vi "DBM Create Proc.vi"(8 "에러 입력":errorcluster, 11 "세부분류번호":string) -> (0 "에러 출력":errorcluster)   [LabVIEW 2020]
uses:
  Variables/Global_Constant.vi
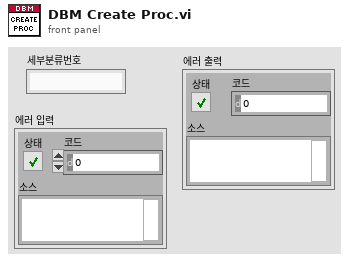
[diagram p1: front panel]
types:
  T1 = enum32{"Invalid", "Default", "Floating", "Floating/Auto-Hide", "Modal"}
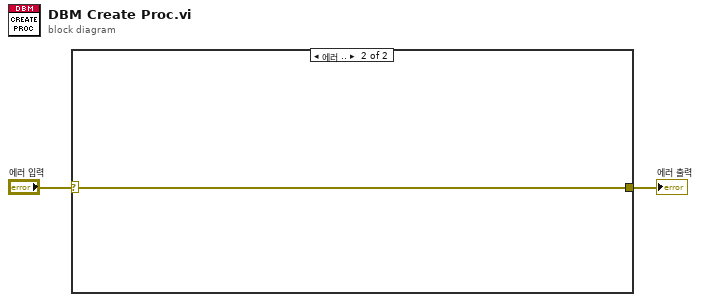
[diagram p0: block diagram]
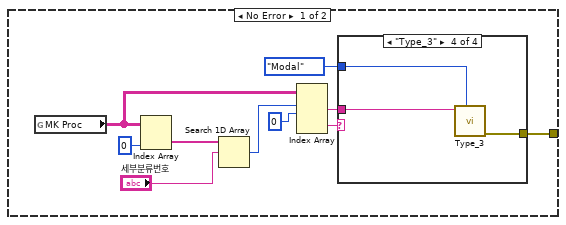
[diagram p2: hidden frame]
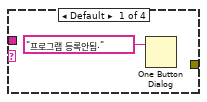
[diagram p3: hidden frame]
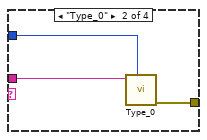
[diagram p4: hidden frame]
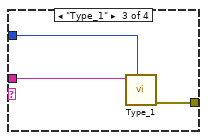
[diagram p5: hidden frame]
diagram:
  n1 = case shown="에러 .." "에러 입력" {
    selector: "에러 입력" -> [_ w23]
    tunnel: [w6 w23] -> w2
    frame No Error {
      n2 = global read "Global_Constant.vi" "MK Proc"() -> (w5:string[][])
      n3 = Index Array(array=w5, index (col)=0 ("비활성화된 인덱스 (열)")) -> (element=w11:string[])  [unwired: 1 in]
      n4 = Search 1D Array(1D array=w11, element="세부분류번호") -> (index of element=w9:i32)  [unwired: 1 in]
      n5 = Index Array(array=w5, index (row) #1=w9, index (col) #1=0 ("비활성화된 인덱스 (열)")) -> (element #1=w7:string, element #2=w4:string)  [unwired: 2 in]
      n6 = case shown="\"Type_3\"" w4 {
        tunnel: w7 -> [_ w16 w19 w22]
        tunnel: [_ w15 w18 w21] -> w6
        tunnel: T1."Modal" ("프런트패널 윈도우:동작") -> [_ w14 w17 w20]
        frame Default {
          n7 = One Button Dialog(message="프로그램 등록안됨." ("메시지")) -> ()  [unwired: 1 in, 1 out]
        }
        frame "Type_0" {
          n8 = call "Type_0.vi"("프런트패널 윈도우:동작"=w14, "세부분류코드"=w16) -> ("error out"=w15:errorcluster)  [unwired: 9 in]
        }
        frame "Type_1" {
          n9 = call "Type_1.vi"("프런트패널 윈도우:동작"=w17, "세부분류코드"=w19) -> ("error out"=w18:errorcluster)  [unwired: 9 in]
        }
        frame "Type_3" {
          n10 = call "Type_3.vi"("프런트패널 윈도우:동작"=w20, "세부분류코드"=w22) -> ("error out"=w21:errorcluster)  [unwired: 9 in]
        }
      }
    }
    frame Error {
    }
  }
  "에러 출력" <- w2
